vi "Server_Main.vi"() -> ()   [LabVIEW 2018, in "Cloud Server.lvlib"]
uses:
  Cloud Server.lvlib
  <vilib>/Platform/TimedLoop/XDataNode/timing_clust.ctl
  <vilib>/Platform/TimedLoop/XDataNode/nitl_modes.ctl
  <vilib>/Platform/TimedLoop/XDataNode/wakeup.ctl
  Data Def/Server_Error Handle Method.ctl
  Data Def/Server_Main Update Data.ctl
  Com VIs/Data Def/Data File Format.ctl
  Data Def/Server_Main Loop Queue Data.ctl
  Data Def/Server_Main Loop State.ctl
  Com VIs/Data Def/User Data.ctl
  Data Def/Server_Connection Manager Method.ctl
  Data Def/Server_Server Write Queue Data.ctl
  <vilib>/Platform/TimedLoop/XDataNode/XDataNode.xnode
  <vilib>/Platform/TimedLoop/XDataNode/XDNodeRunTimeDep.lvlib
panel:
  out "Number Of Connections":i32
  in  "Tab Control":T1(tab)
  out "User Data":T2 {"Last Login Time" format="%<%x %.3X>T"}
  out "Remote Data":waveform(dbl)(graph)
  out "User Picture":T3(plugin-control)
  in  "Scrollbar":i32(c297)
  out "Training Result":string
  out "Training Data":waveform(dbl)(graph)
  in  "Data Query List":i32(listbox)
  out "Query Data":waveform(dbl)(graph)
  in  "User Name List":i32(listbox)=-1
  # "Smart ECG Server"
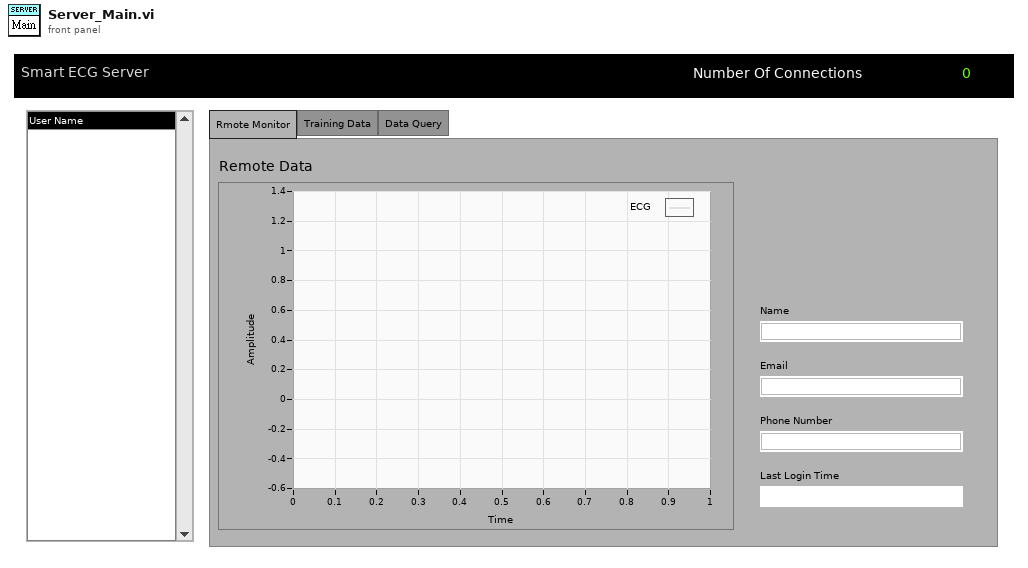
[diagram p1: front panel]
types:
  T1 = enum32{"Rmote Monitor", "Training Data", "Data Query"}
  T2 = cluster{"Name":string, "Email":string, "Phone Number":string, "Last Login Time":timestamp}
  T3 = typedef "IMAQ Image.ctl" = refnum<image>
  T4 = typedef "XDNodeRunTimeDep.lvlib/timing_clust.ctl" = cluster{"Expected End [f-1]":u64, "Actual End [f-1]":u64, "Finished Late? [f-1]":bool, "Expected End [i-1]":u64, "Actual End [i-1]":u64, "Finished Late? [i-1]":bool, "Expected Start [i]":u64, "Actual Start [i]":u64, "Expected Start [f]":u64, "Actual Start [f]":u64, "Source Name":string, "Structure Name":string, "Period":i64, "Deadline":i64, "Offset":i64, "Start":i64, "Priority":i32, "Timeout":i32, "Mode":T5, "Wakeup Reason":T6, "Error":errorcluster, "Source Type":string, "Secondary Source Type":string, "Global End Time":u64, "Global Start Time":u64, "Frame Duration":u64, "Iteration Duration":u64, "Assigned CPU":i32, "I/O Scan Engine Mode":u32}
  T5 = typedef "XDNodeRunTimeDep.lvlib/nitl_modes.ctl" = enum32{"No Change", "Process missed periods, maintain original phase", "Discard missed periods, maintain original phase", "Process missed periods, ignore original phase", "Discard missed periods, ignore original phase"}
  T6 = typedef "XDNodeRunTimeDep.lvlib/wakeup.ctl" = enum32{"Normal", "Aborted", "Asynchronous wakeup", "Timing source error", "Timed loop error", "Timeout"}
  T7 = typedef "Cloud Server.lvlib/Server_Main Loop Queue Data.ctl" = cluster{"Main Loop State":T8, "Data":variant}
  T8 = typedef "Cloud Server.lvlib/Server_Main Loop State.ctl" = enum16{"Detect", "Save", "Training", "Refresh User Name", "Stop"}
  T9 = typedef "User Data.ctl" = cluster{"Name":string, "Email":string, "Phone Number":string, "User Picture":u32[][], "Last Login Time":timestamp}
  T10 = typedef "Cloud Server.lvlib/Server_Main Data.ctl" = cluster{"Main VI Ref.":refnum<vi>, "Listener ID":refnum<k5>, "Meta data":T11[], "Main Queue":T13, "User Picture":T3}
  T11 = typedef "stm_MetaElement.ctl" = cluster{"Name":T12}
  T12 = typedef "stm_MetaDataElement.ctl" = string
  T13 = typedef "Cloud Server.lvlib/Server_Main Queue.ctl" = cluster{"Server Write Queue":refnum<queue>, "Main Loop Queue":refnum<queue>}
  T14 = typedef "Cloud Server.lvlib/Server_Server Write Queue Data.ctl" = cluster{"connection ID":refnum<k5>, "Meta Data":string, "Data":variant}
  T15 = typedef "User Registering Status.ctl" = enum16{"Failed", "Duplicate", "Success"}
  T16 = typedef "Cloud Server.lvlib/Server_Error Handle Method.ctl" = enum16{"Initialize", "Get Queue Ref.", "Enqueue", "Insert", "Flush", "Release"}
  T17 = typedef "Cloud Server.lvlib/Server_Connection Manager Method.ctl" = enum16{"Initialize", "Add", "Get", "Set Properties", "Get Properties", "Close", "Release"}
  T18 = typedef "Cloud Server.lvlib/Server_Main Update Data.ctl" = cluster{"Data":waveform(dbl), "connection ID":refnum<k5>}
  T19 = typedef "Cloud Server.lvlib/Server_Connection Properties.ctl" = cluster{"User Data":T9, "Data":waveform(dbl)}
  T20 = typedef "Data File Format.ctl" = cluster{"Data":waveform(dbl), "Abnormal?":bool, "Measure Time":timestamp, "User Name":string}
  T21 = typedef "Cloud Server.lvlib/Server_Training Data.ctl" = cluster{"Data":waveform(dbl), "Abnormal?":bool}
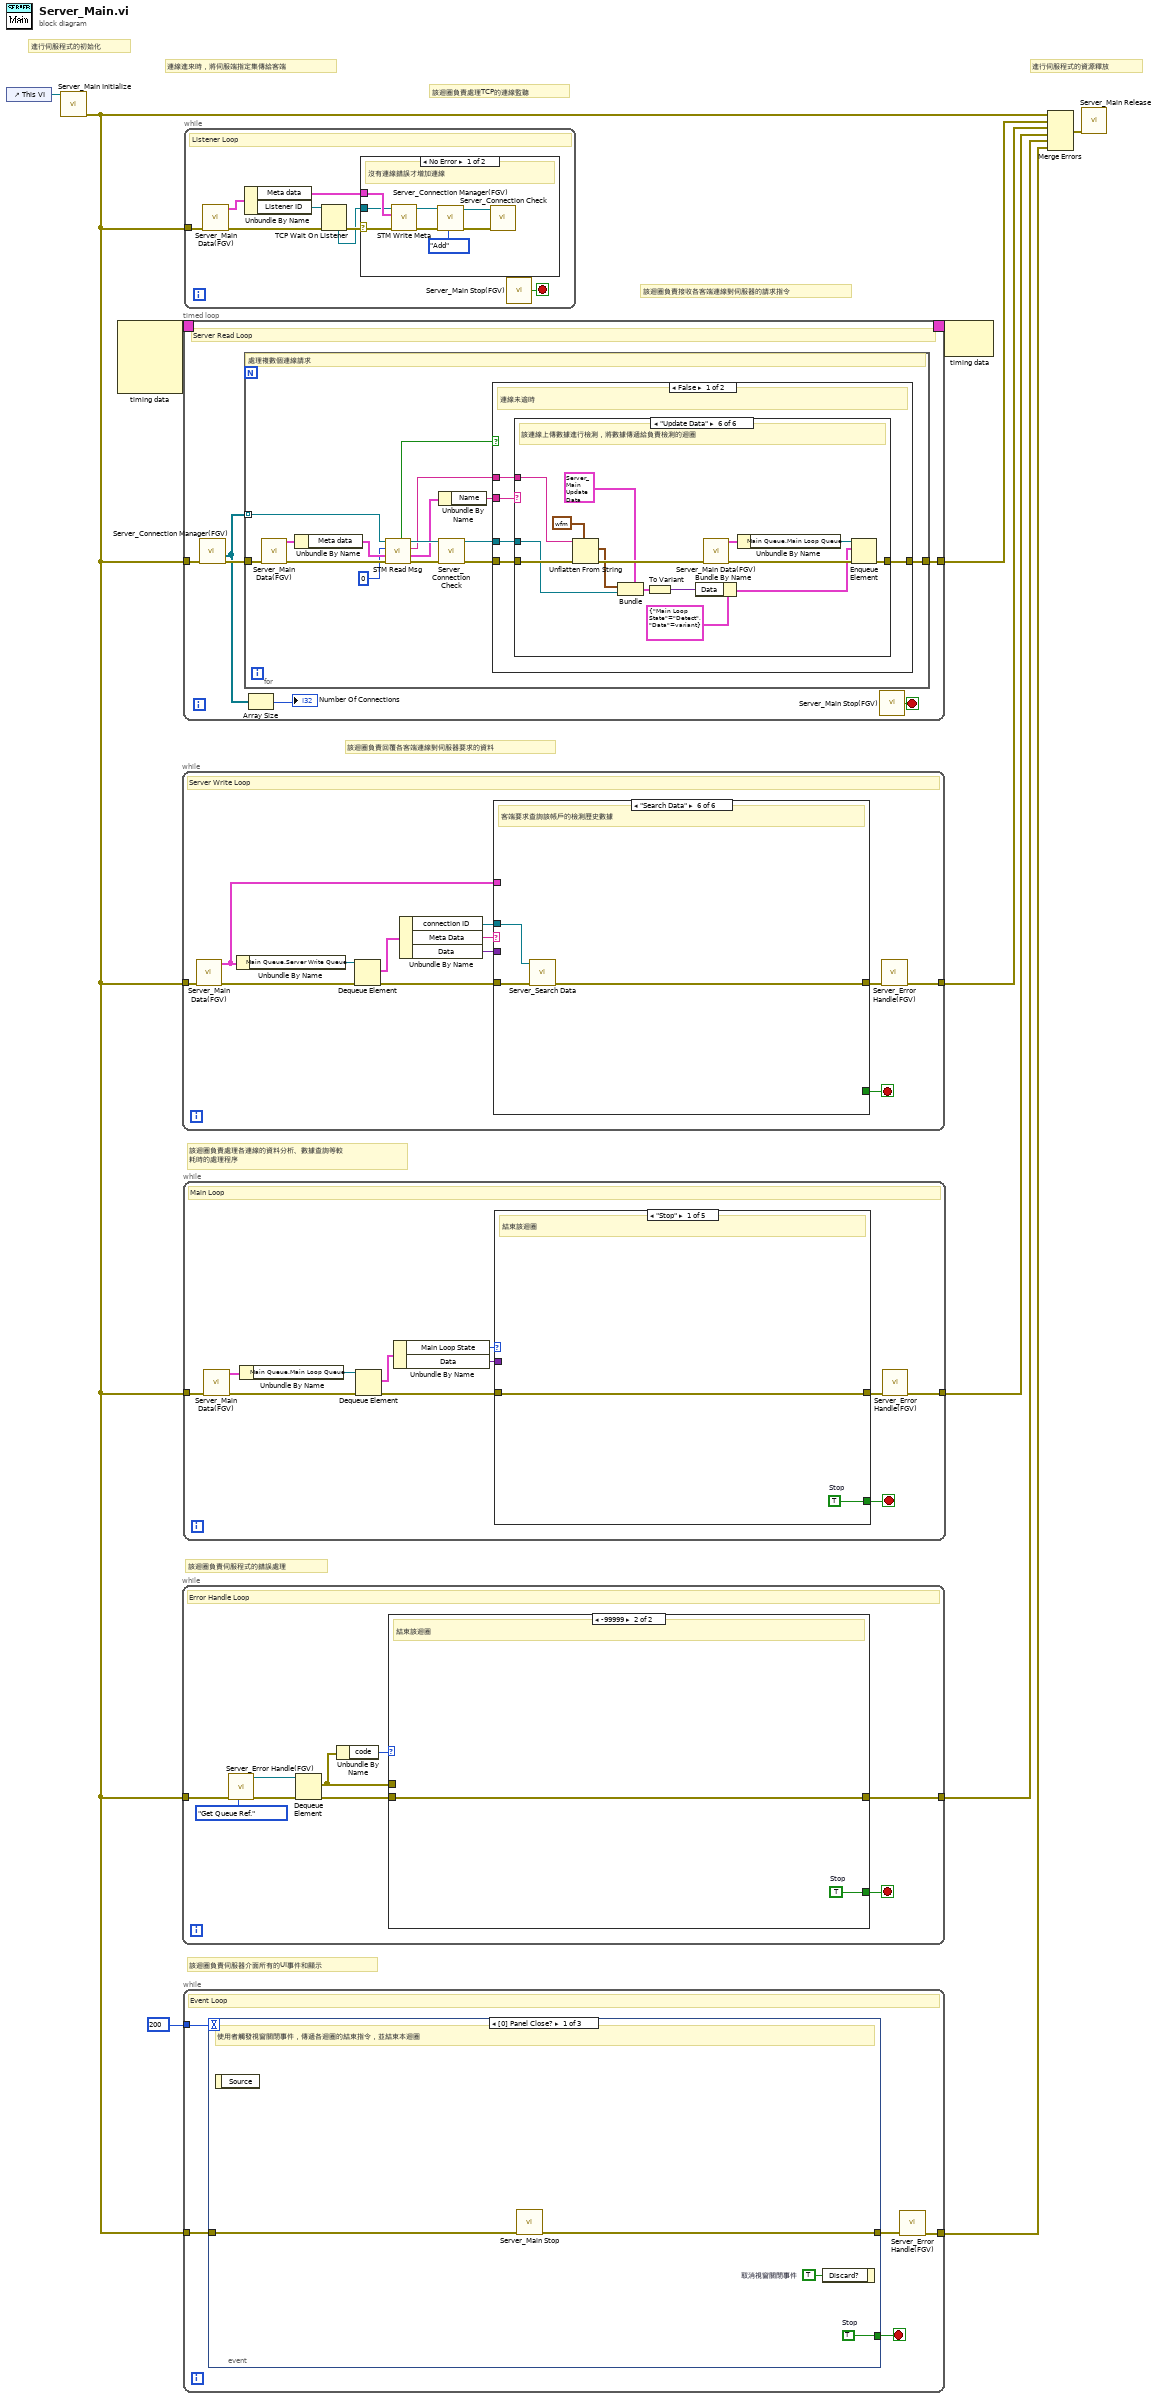
[diagram p0: block diagram]
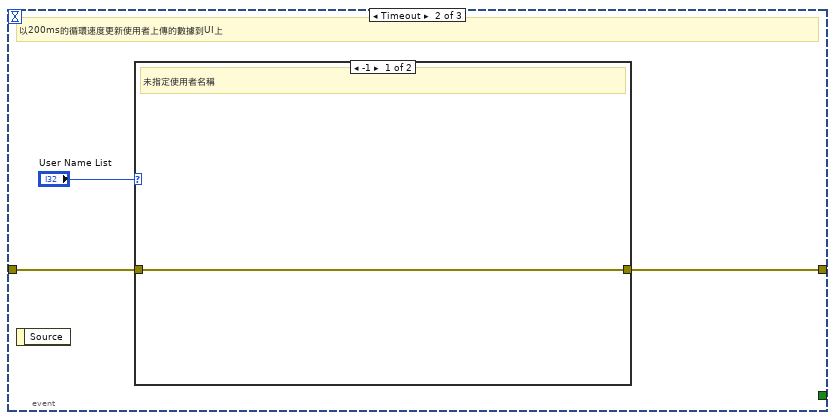
[diagram p2: hidden frame]
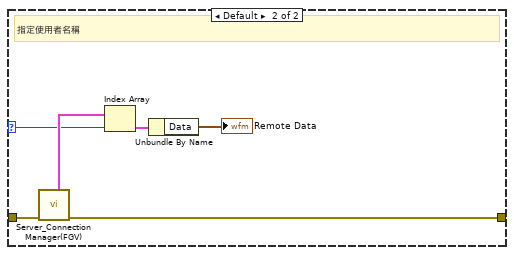
[diagram p3: hidden frame]
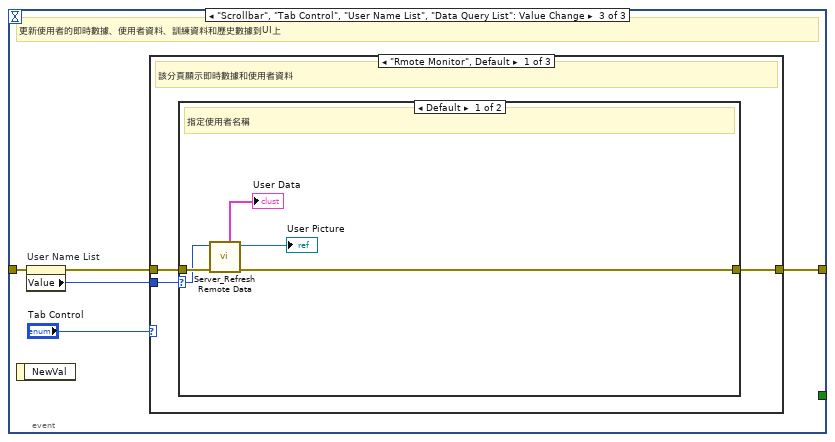
[diagram p4: hidden frame]
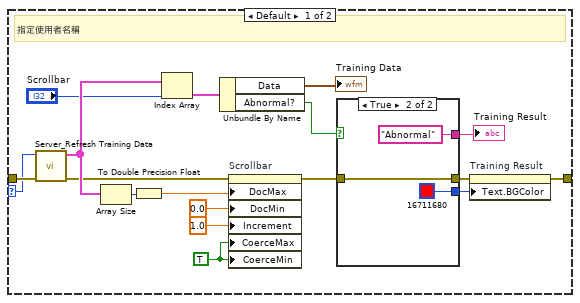
[diagram p7: hidden frame]
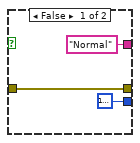
[diagram p8: hidden frame]
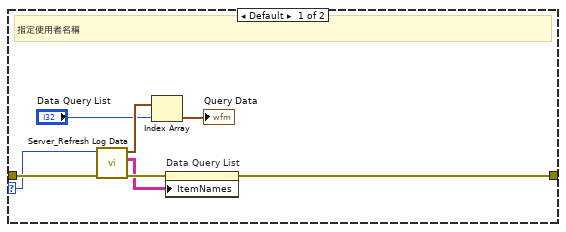
[diagram p10: hidden frame]
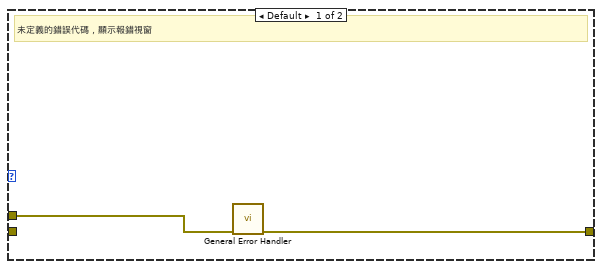
[diagram p11: hidden frame]
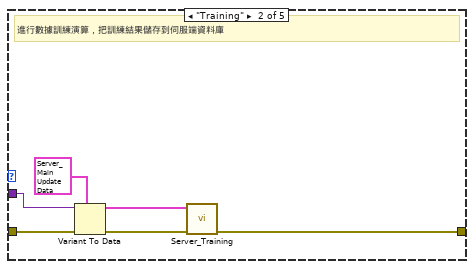
[diagram p12: hidden frame]
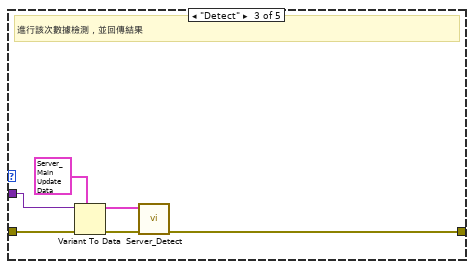
[diagram p13: hidden frame]
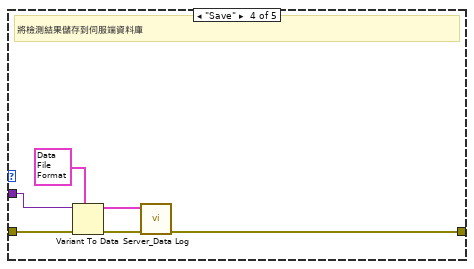
[diagram p14: hidden frame]
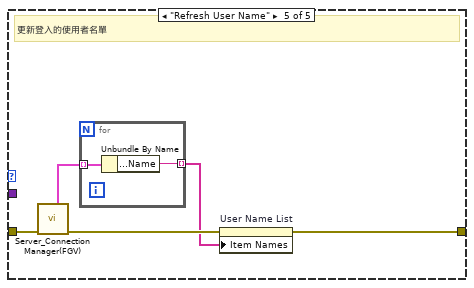
[diagram p15: hidden frame]
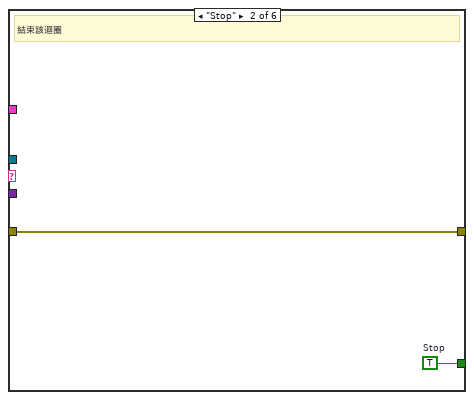
[diagram p17: hidden frame]
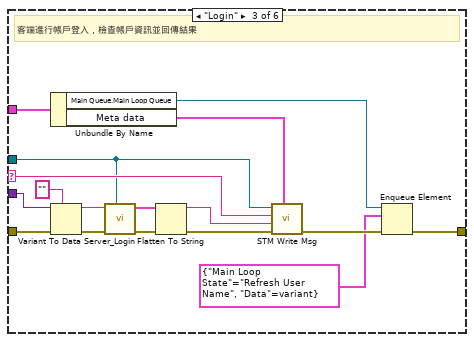
[diagram p18: hidden frame]
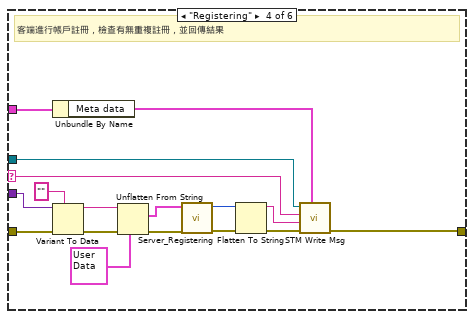
[diagram p19: hidden frame]
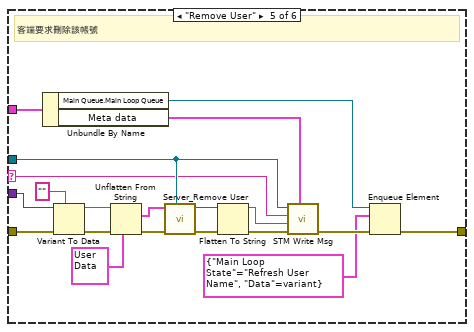
[diagram p20: hidden frame]
diagram:
  # "連線進來時，將伺服端指定集傳給客端"
  # "進行伺服程式的資源釋放"
  # "進行伺服程式的初始化"
  # "該迴圈負責伺服器介面所有的UI事件和顯示"
  # "該迴圈負責伺服程式的錯誤處理"
  # "該迴圈負責處理各連線的資料分析、數據查詢等較\n耗時的處理程序"
  # "該迴圈負責回覆各客端連線對伺服器要求的資料"
  # "該迴圈負責接收各客端連線對伺服器的請求指令"
  # "該迴圈負責處理TCP的連線監聽"
  n1 = control-ref of="This VI"() -> (w11:refnum<vi>)
  n2 = call "Server_Main Initialize.vi"("VI Reference"=w11) -> ("error out"=w3:errorcluster)  [unwired: 10 in]
  n3 = node-c288() -> (w10:T4)  [unwired: 4 in]
  n4 = while {
    tunnel: w3 -> [w23]
    tunnel: [w15] -> w6
    stop <- w13 stop-if-true
    # "Server Write Loop"
    n5 = call "Server_Main Data(FGV).vi"("error in"=w23) -> ("error out"=w22:errorcluster, "Main Data Out"=w12:T10)  [unwired: 9 in]
    n6 = Unbundle By Name(w12) -> ("Main Queue.Server Write Queue"=w21:refnum<queue>)
    n7 = Dequeue Element(queue=w21, error in (no error)=w22) -> (element=w20:T14, error out=w19:errorcluster)  [unwired: 1 in, 2 out]
    n8 = Unbundle By Name(w20) -> ("connection ID"=w16:refnum<k5>, "Meta Data"=w18:string, "Data"=w17:variant)
    n9 = case shown="\"Search Data\"" w18 {
      selector: w18 -> [_ _ w32 w51 w66 _]
      tunnel: w19 -> [w24 w26 w43 w60 w76 w83]
      tunnel: w17 -> [_ _ w42 w59 w75 _]
      tunnel: w16 -> [_ _ w31 w44 w68 w82]
      tunnel: [w24 w26 w29 w55 w63 w81] -> w14
      tunnel: [_ w25 _ _ _ _] -> w13
      tunnel: w12 -> [_ _ w38 w54 w70 _]
      frame Default {
        # "忽略，未定義的命令"
      }
      frame "Stop" {
        w25 = TRUE  # Stop
        # "結束該迴圈"
      }
      frame "Login" {
        # "客端進行帳戶登入，檢查帳戶資訊並回傳結果"
        n10 = Unbundle By Name(w38) -> ("Main Queue.Main Loop Queue"=w28:refnum<queue>, "Meta data"=w34:T11[])
        n11 = Variant To Data(error in=w43, type="", Variant=w42) -> (data=w39:string, error out=w40:errorcluster)
        n12 = call "Server_Login.vi"("connection ID"=w31, "error in"=w40, "User Name"=w39) -> ("error out"=w37:errorcluster, "User Data"=w36:T9)  [unwired: 7 in]
        n13 = Flatten To String(anything=w36, error in (no error)=w37) -> (data string=w33:string, error out=w35:errorcluster)  [unwired: 2 in, 1 out]
        n14 = call "STM Write Msg.vi"("Meta data"=w34, "error in (no error)"=w35, "Data"=w33, "Name"=w32, "connection ID"=w31) -> ("error out"=w30:errorcluster)  [unwired: 5 in, 1 out]
        n15 = Enqueue Element(queue=w28, element=T7 {"Main Loop State"=enum."Refresh User Name", "Data"=variant}, error in (no error)=w30) -> (error out=w29:errorcluster)  [unwired: 1 in, 2 out]
      }
      frame "Registering" {
        # "客端進行帳戶註冊，檢查有無重複註冊，並回傳結果"
        n16 = Unbundle By Name(w54) -> ("Meta data"=w53:T11[])
        n17 = Variant To Data(error in=w60, type="", Variant=w59) -> (data=w48:string, error out=w49:errorcluster)
        n18 = Unflatten From String(type=T9 {"Name"="Guset", "Email"="", "Phone Number"="", "User Picture"=array225x225[50625 elements], "Last Login Time"=timestamp(0 s since 1904-01-01)} ("User Data"), binary string=w48, error in (no error)=w49) -> (value=w45:T9, error out=w46:errorcluster)  [unwired: 2 in, 1 out]
        n19 = call "Server_Registering.vi"("error in"=w46, "User Data"=w45) -> ("error out"=w58:errorcluster, "User Registering Status"=w57:T15)  [unwired: 8 in]
        n20 = Flatten To String(anything=w57, error in (no error)=w58) -> (data string=w52:string, error out=w56:errorcluster)  [unwired: 2 in, 1 out]
        n21 = call "STM Write Msg.vi"("Meta data"=w53, "error in (no error)"=w56, "Data"=w52, "Name"=w51, "connection ID"=w44) -> ("error out"=w55:errorcluster)  [unwired: 5 in, 1 out]
      }
      frame "Remove User" {
        # "客端要求刪除該帳號"
        n22 = Unbundle By Name(w70) -> ("Main Queue.Main Loop Queue"=w62:refnum<queue>, "Meta data"=w69:T11[])
        n23 = Variant To Data(error in=w76, type="", Variant=w75) -> (data=w78:string, error out=w79:errorcluster)
        n24 = Unflatten From String(type=T9 {"Name"="Guset", "Email"="", "Phone Number"="", "User Picture"=array225x225[50625 elements], "Last Login Time"=timestamp(0 s since 1904-01-01)} ("User Data"), binary string=w78, error in (no error)=w79) -> (value=w73:T9, error out=w74:errorcluster)  [unwired: 2 in, 1 out]
        n25 = call "Server_Remove User.vi"("connection ID"=w68, "error in"=w74, "User Data"=w73) -> ("error out"=w72:errorcluster, "OK?"=w71:bool)  [unwired: 7 in]
        n26 = Flatten To String(anything=w71, error in (no error)=w72) -> (data string=w65:string, error out=w67:errorcluster)  [unwired: 2 in, 1 out]
        n27 = call "STM Write Msg.vi"("Meta data"=w69, "error in (no error)"=w67, "Data"=w65, "Name"=w66, "connection ID"=w68) -> ("error out"=w64:errorcluster)  [unwired: 5 in, 1 out]
        n28 = Enqueue Element(queue=w62, element=T7 {"Main Loop State"=enum."Refresh User Name", "Data"=variant}, error in (no error)=w64) -> (error out=w63:errorcluster)  [unwired: 1 in, 2 out]
      }
      frame "Search Data" {
        # "客端要求查詢該帳戶的檢測歷史數據"
        n29 = call "Server_Search Data.vi"("error in"=w83, "connection ID"=w82) -> ("error out"=w81:errorcluster)  [unwired: 9 in]
      }
    }
    n30 = call "Server_Error Handle(FGV).vi"("error in"=w14) -> ("error out"=w15:errorcluster)  [unwired: 9 in, 1 out]
  }
  n31 = while {
    tunnel: w3 -> [w90]
    tunnel: [w85] -> w4
    stop <- w91 stop-if-true
    # "Error Handle Loop"
    n32 = call "Server_Error Handle(FGV).vi"("Error Handle Method(Enqueue)"=Server_Error_Handle_Method."Get Queue Ref.", "error in"=w90) -> ("error out"=w89:errorcluster, "Queue Ref."=w87:refnum<queue>)  [unwired: 8 in]
    n33 = Dequeue Element(queue=w87, error in (no error)=w89) -> (element=w84:errorcluster, error out=w92:errorcluster)  [unwired: 1 in, 2 out]
    n34 = Unbundle By Name(w84) -> ("code"=w86:i32)
    n35 = case shown="-99999" w86 {
      tunnel: w92 -> [_ w95]
      tunnel: [w94 w95] -> w85
      tunnel: [_ w96] -> w91
      tunnel: w84 -> [w93 _]
      frame Default {
        # "未定義的錯誤代碼，顯示報錯視窗"
        n36 = call <vilib>:"General Error Handler.vi"("error in (no error)"=w93) -> ("error out"=w94:errorcluster)  [unwired: 10 in, 4 out]
      }
      frame -99999 {
        w96 = TRUE  # Stop
        # "結束該迴圈"
      }
    }
  }
  n37 = timed-loop {
    tunnel: w3 -> [w102]
    timing: w10 -> [_]
    timing-out: [_] -> w9
    tunnel: [w99] -> w8
    stop <- w100 stop-if-true
    # "Server Read Loop"
    n38 = call "Server_Connection Manager(FGV).vi"("error in"=w102) -> ("error out"=w101:errorcluster, "All Connections"=w98:refnum<k5>[])  [unwired: 6 in, 3 out]
    n39 = for {
      tunnel: w101 -> [w114]
      tunnel: w98 -> [w117] mode=indexing
      tunnel: [w104] -> w99
      # "處理複數個連線請求"
      n40 = call "Server_Main Data(FGV).vi"("error in"=w114) -> ("error out"=w112:errorcluster, "Main Data Out"=w113:T10)  [unwired: 9 in]
      n41 = Unbundle By Name(w113) -> ("Meta data"=w111:T11[])
      n42 = call "STM Read Msg.vi"("error in"=w112, "Meta data"=w111, "timeout ms (25000)"=0, "connection ID"=w117) -> ("error out"=w116:errorcluster, "Meta element"=w106:T11, "data string"=w107:string, "connection ID out"=w115:refnum<k5>, "Timed Out?"=w103:bool)  [unwired: 2 in, 1 out]
      n43 = Unbundle By Name(w106) -> ("Name"=w105:T12)
      n44 = call "Server_Connection Check.vi"("error in"=w116, "Connection In"=w115) -> ("error out"=w109:errorcluster, "Connection out"=w108:refnum<k5>)  [unwired: 7 in, 1 out]
      n45 = case shown="False" w103 {
        tunnel: w109 -> [w120 w187]
        tunnel: w108 -> [w118 _]
        tunnel: w107 -> [w122 _]
        tunnel: w105 -> [w121 _]
        tunnel: [w119 w187] -> w104
        frame False {
          # "連線未逾時"
          n46 = case shown="\"Update Data\"" w121 {
            selector: w121 -> [_ w127 _ _ _ _]
            tunnel: w122 -> [_ w129 _ w155 w169 w184]
            tunnel: w120 -> [w123 w134 w143 w156 w170 w185]
            tunnel: [w123 w124 w136 w145 w164 w179] -> w119
            tunnel: w118 -> [_ w126 w141 w152 w167 w182]
            frame Default {
              # "忽略，未定義的命令"
            }
            frame "Login", "Registering", "Remove User", "Search Data" {
              # "把請求傳遞到負責TCP回復資料的迴圈"
              n47 = To Variant(anything=w129) -> (Variant=w128:variant)
              n48 = call "Server_Main Data(FGV).vi"("error in"=w134) -> ("error out"=w132:errorcluster, "Main Data Out"=w133:T10)  [unwired: 9 in]
              n49 = Unbundle By Name(w133) -> ("Main Queue.Server Write Queue"=w131:refnum<queue>)
              n50 = Bundle By Name(cluster=T14 {"connection ID"=refnum, "Meta Data"="", "Data"=variant} ("element"), "Data"=w128, "Meta Data"=w127, "connection ID"=w126) -> (w125:T14)
              n51 = Enqueue Element(queue=w131, element=w125, error in (no error)=w132) -> (error out=w124:errorcluster)  [unwired: 1 in, 2 out]
            }
            frame "Logout" {
              # "該連線進行登出"
              n52 = call "Server_Connection Manager(FGV).vi"("Connection Manager Method(Get)"=Server_Connection_Manager_Method."Close", "error in"=w143, "Connection In"=w141) -> ("error out"=w140:errorcluster)  [unwired: 4 in, 4 out]
              n53 = call "Server_Main Data(FGV).vi"("error in"=w140) -> ("error out"=w138:errorcluster, "Main Data Out"=w139:T10)  [unwired: 9 in]
              n54 = Unbundle By Name(w139) -> ("Main Queue.Main Loop Queue"=w137:refnum<queue>)
              n55 = Enqueue Element(queue=w137, element=T7 {"Main Loop State"=enum."Refresh User Name", "Data"=variant}, error in (no error)=w138) -> (error out=w136:errorcluster)  [unwired: 1 in, 2 out]
            }
            frame "Live Mode" {
              # "該連線連續上傳資料"
              n56 = Unflatten From String(type=waveform(dbl) {"t0"=timestamp(0 s since 1904-01-01), "dt"=1.0, "Y"=[]} ("waveform"), binary string=w155, error in (no error)=w156) -> (value=w146:waveform(dbl), error out=w153:errorcluster)  [unwired: 2 in, 1 out]
              n57 = call "Server_Connection Manager(FGV).vi"("Connection Manager Method(Get)"=Server_Connection_Manager_Method."Get Properties", "error in"=w153, "Connection In"=w152) -> ("error out"=w150:errorcluster, "Connection Properties Out"=w147:T19, "Connection Out"=w149:refnum<k5>)  [unwired: 4 in, 2 out]
              n58 = Bundle By Name(cluster=w147, "Data"=w146) -> (w144:T19)
              n59 = call "Server_Connection Manager(FGV).vi"("Connection Manager Method(Get)"=Server_Connection_Manager_Method."Set Properties", "error in"=w150, "Connection Properties In"=w144, "Connection In"=w149) -> ("error out"=w145:errorcluster)  [unwired: 3 in, 4 out]
            }
            frame "Training" {
              # "該連線進行訓練演算，將資料傳遞給負責演算的迴圈"
              n60 = Unflatten From String(type=waveform(dbl) {"t0"=timestamp(0 s since 1904-01-01), "dt"=1.0, "Y"=[]} ("Data"), binary string=w169, error in (no error)=w170) -> (value=w157:waveform(dbl), error out=w168:errorcluster)  [unwired: 2 in, 1 out]
              n61 = Bundle(cluster=T18 {"Data"={"t0"=timestamp(0 s since 1904-01-01), "dt"=1.0, "Y"=[]}, "connection ID"=refnum} ("Main Training Data"), "Data"=w157, "connection ID"=w167) -> (w163:T18)
              n62 = To Variant(anything=w163) -> (Variant=w162:variant)
              n63 = Bundle By Name(cluster=T7 {"Main Loop State"=enum."Training", "Data"=variant} ("element"), "Data"=w162) -> (w160:T7)
              n64 = call "Server_Main Data(FGV).vi"("error in"=w168) -> ("error out"=w166:errorcluster, "Main Data Out"=w171:T10)  [unwired: 9 in]
              n65 = Unbundle By Name(w171) -> ("Main Queue.Main Loop Queue"=w165:refnum<queue>)
              n66 = Enqueue Element(queue=w165, element=w160, error in (no error)=w166) -> (error out=w164:errorcluster)  [unwired: 1 in, 2 out]
            }
            frame "Update Data" {
              # "該連線上傳數據進行檢測，將數據傳遞給負責檢測的迴圈"
              n67 = Unflatten From String(type=waveform(dbl) {"t0"=timestamp(0 s since 1904-01-01), "dt"=1.0, "Y"=[]} ("Data"), binary string=w184, error in (no error)=w185) -> (value=w172:waveform(dbl), error out=w183:errorcluster)  [unwired: 2 in, 1 out]
              n68 = Bundle(cluster=T18 {"Data"={"t0"=timestamp(0 s since 1904-01-01), "dt"=1.0, "Y"=[]}, "connection ID"=refnum} ("Main Training Data"), "Data"=w172, "connection ID"=w182) -> (w178:T18)
              n69 = To Variant(anything=w178) -> (Variant=w177:variant)
              n70 = Bundle By Name(cluster=T7 {"Main Loop State"=enum."Detect", "Data"=variant} ("element"), "Data"=w177) -> (w175:T7)
              n71 = call "Server_Main Data(FGV).vi"("error in"=w183) -> ("error out"=w181:errorcluster, "Main Data Out"=w186:T10)  [unwired: 9 in]
              n72 = Unbundle By Name(w186) -> ("Main Queue.Main Loop Queue"=w180:refnum<queue>)
              n73 = Enqueue Element(queue=w180, element=w175, error in (no error)=w181) -> (error out=w179:errorcluster)  [unwired: 1 in, 2 out]
            }
          }
        }
        frame True {
          # "逾時，沒收到請求"
        }
      }
    }
    n74 = Array Size(array=w98) -> (size(s)=→"Number Of Connections":i32)
    n75 = call "Server_Main Stop(FGV).vi"() -> ("Stop Out"=w100:bool)  [unwired: 4 in]
  }
  n76 = while {
    tunnel: w3 -> [w200]
    tunnel: [w192] -> w5
    stop <- w190 stop-if-true
    # "Main Loop"
    n77 = call "Server_Main Data(FGV).vi"("error in"=w200) -> ("error out"=w198:errorcluster, "Main Data Out"=w199:T10)  [unwired: 9 in]
    n78 = Unbundle By Name(w199) -> ("Main Queue.Main Loop Queue"=w197:refnum<queue>)
    n79 = Dequeue Element(queue=w197, error in (no error)=w198) -> (element=w196:T7, error out=w195:errorcluster)  [unwired: 1 in, 2 out]
    n80 = Unbundle By Name(w196) -> ("Main Loop State"=w194:T8, "Data"=w193:variant)
    n81 = case shown="\"Stop\"" w194 {
      tunnel: w195 -> [w202 w208 w214 w220 w225]
      tunnel: w193 -> [_ w207 w213 w219 _]
      tunnel: [w202 w204 w209 w217 w221] -> w191
      tunnel: [w201 _ _ _ _] -> w190
      frame "Stop" {
        w201 = TRUE  # Stop
        # "結束該迴圈"
      }
      frame "Training" {
        # "進行數據訓練演算，把訓練結果儲存到伺服端資料庫"
        n82 = Variant To Data(error in=w208, type=T18 {"Data"={"t0"=timestamp(0 s since 1904-01-01), "dt"=1.0, "Y"=[]}, "connection ID"=refnum} ("Main Training Data"), Variant=w207) -> (data=w203:T18, error out=w205:errorcluster)
        n83 = call "Server_Training.vi"("error in"=w205, "Main Update Data"=w203) -> ("error out"=w204:errorcluster)  [unwired: 9 in]
      }
      frame "Detect" {
        # "進行該次數據檢測，並回傳結果"
        n84 = Variant To Data(error in=w214, type=T18 {"Data"={"t0"=timestamp(0 s since 1904-01-01), "dt"=1.0, "Y"=[]}, "connection ID"=refnum} ("Main Training Data"), Variant=w213) -> (data=w210:T18, error out=w211:errorcluster)
        n85 = call "Server_Detect.vi"("error in"=w211, "Main Update Data"=w210) -> ("error out"=w209:errorcluster)  [unwired: 9 in]
      }
      frame "Save" {
        # "將檢測結果儲存到伺服端資料庫"
        n86 = Variant To Data(error in=w220, type=T20 {"Data"={"t0"=timestamp(0 s since 1904-01-01), "dt"=1.0, "Y"=[]}, "Abnormal?"=FALSE, "Measure Time"=timestamp(0 s since 1904-01-01), "User Name"=""} ("Data File Format"), Variant=w219) -> (data=w216:T20, error out=w218:errorcluster)
        n87 = call "Server_Data Log.vi"("error in"=w218, "Data File Format"=w216) -> ("error out"=w217:errorcluster)  [unwired: 9 in]
      }
      frame "Refresh User Name" {
        # "更新登入的使用者名單"
        n88 = call "Server_Connection Manager(FGV).vi"("error in"=w225) -> ("error out"=w223:errorcluster, "All Connection Properties"=w224:T19[])  [unwired: 6 in, 3 out]
        n89 = for {
          tunnel: w224 -> [w227] mode=indexing
          tunnel: [w226] -> w222 mode=indexing
          n90 = Unbundle By Name(w227) -> ("User Data.Name"=w226:string)
        }
        n91 = property on="User Name List" class="LstBox (strict)"(error in=w223, "Item Names"=w222) -> (error out=w221:errorcluster)  [unwired: 1 in, 1 out]
      }
    }
    n92 = call "Server_Error Handle(FGV).vi"("error in"=w191) -> ("error out"=w192:errorcluster)  [unwired: 9 in, 1 out]
  }
  n93 = while {
    tunnel: w3 -> [w232]
    tunnel: [w231] -> w2
    tunnel: 200 -> [w228]
    stop <- w230 stop-if-true
    # "Event Loop"
    n94 = event shown="[0] Panel Close?" {
      selector: _ -> [_ _ _]
      dyn-events: _ -> [_ _ _]
      timeout: w228 -> [_ _ _]
      tunnel: w232 -> [w234 w239 w250]
      tunnel: [w236 _ _] -> w230
      tunnel: [w233 w237 w247] -> w229
      event Panel Close? {
        w235 = TRUE  # 取消視窗關閉事件
        w236 = TRUE  # Stop
        # "使用者觸發視窗關閉事件，傳遞各迴圈的結束指令，並結束本迴圈"
        n95 = event-data() -> ()  [unwired: 1 in, 1 out]
        n96 = call "Server_Main Stop.vi"("error in"=w234) -> ("error out"=w233:errorcluster)  [unwired: 10 in]
        n97 = event-data("Discard?"=w235) -> ()  [unwired: 1 in, 1 out]
      }
      event Timeout {
        # "以200ms的循環速度更新使用者上傳的數據到UI上"
        n98 = event-data() -> ()  [unwired: 1 in, 1 out]
        n99 = case shown="-1" "User Name List" {
          selector: "User Name List" -> [_ w244]
          tunnel: w239 -> [w240 w246]
          tunnel: [w240 w242] -> w237
          frame -1 {
            # "未指定使用者名稱"
          }
          frame Default {
            # "指定使用者名稱"
            n100 = call "Server_Connection Manager(FGV).vi"("error in"=w246) -> ("error out"=w242:errorcluster, "All Connection Properties"=w245:T19[])  [unwired: 6 in, 3 out]
            n101 = Index Array(array=w245, index=w244) -> (element=w243:T19)
            n102 = Unbundle By Name(w243) -> ("Data"=→"Remote Data":waveform(dbl))
          }
        }
      }
      event "Scrollbar", "Tab Control", "User Name List", "Data Query List": Value Change {
        # "更新使用者的即時數據、使用者資料、訓練資料和歷史數據到UI上"
        n103 = event-data() -> ()  [unwired: 1 in, 1 out]
        n104 = property on="User Name List" class="LstBox (strict)"(error in=w250) -> (error out=w249:errorcluster, "Value"=w248:i32)  [unwired: 1 in, 1 out]
        n105 = case shown="\"Rmote Monitor\", Default" "Tab Control" {
          tunnel: w249 -> [w253 w262 w291]
          tunnel: w248 -> [w254 w263 w290]
          tunnel: [w252 w261 w289] -> w247
          frame "Rmote Monitor", Default {
            # "該分頁顯示即時數據和使用者資料"
            n106 = case shown="Default" w254 {
              selector: w254 -> [w255 _]
              tunnel: w253 -> [w257 w260]
              tunnel: [w256 w260] -> w252
              frame Default {
                # "指定使用者名稱"
                n107 = call "Server_Refresh Remote Data.vi"("error in"=w257, "Index"=w255) -> ("error out"=w256:errorcluster, "Image"=→"User Picture":T3, "User Data"=→"User Data":T2)  [unwired: 7 in]
              }
              frame -1 {
                # "未指定使用者名稱"
              }
            }
          }
          frame "Training Data" {
            # "該分頁顯示使用者的訓練資料"
            n108 = case shown="-1" w263 {
              selector: w263 -> [w280 _]
              tunnel: w262 -> [w281 w288]
              tunnel: [w275 w288] -> w261
              frame Default {
                w264 = TRUE ("Coerce Minimum Value")
                # "指定使用者名稱"
                n109 = call "Server_Refresh Training Data.vi"("error in"=w281, "Index"=w280) -> ("error out"=w269:errorcluster, "Training Data"=w278:T21[])  [unwired: 8 in]
                n110 = Array Size(array=w278) -> (size(s)=w279:i32)
                n111 = To Double Precision Float(number=w279) -> (double precision float=w267:dbl)
                n112 = Index Array(array=w278, index="Scrollbar") -> (element=w277:T21)
                n113 = Unbundle By Name(w277) -> ("Data"=→"Training Data":waveform(dbl), "Abnormal?"=w274:bool)
                n114 = property on="Scrollbar" class="Scroll (strict)"(error in=w269, "DocMax"=w267, "DocMin"=0.0 ("Scale.Range:Minimum"), "Increment"=1.0, "CoerceMax"=w264, "CoerceMin"=w264) -> (error out=w268:errorcluster)  [unwired: 1 in, 1 out]
                n115 = case shown="True" w274 {
                  tunnel: w268 -> [w284 w287]
                  tunnel: [w284 w287] -> w273
                  tunnel: [u32 16777216 u32 16711680] -> w272
                  tunnel: ["Normal" "Abnormal"] -> w271
                  frame False {
                  }
                  frame True {
                  }
                }
                "Training Result" <- w271
                n116 = property on="Training Result" class="Str"(error in=w273, "Text.BGColor"=w272) -> (error out=w275:errorcluster)  [unwired: 1 in, 1 out]
              }
              frame -1 {
                # "未指定使用者名稱"
              }
            }
          }
          frame "Data Query" {
            # "該分頁顯示使用者的檢測歷史數據"
            n117 = case shown="-1" w290 {
              selector: w290 -> [w298 _]
              tunnel: w291 -> [w299 w300]
              tunnel: [w296 w300] -> w289
              frame Default {
                # "指定使用者名稱"
                n118 = call "Server_Refresh Log Data.vi"("error in"=w299, "Index"=w298) -> ("error out"=w297:errorcluster, "Data Query List"=w295:string[][], "Data"=w294:waveform(dbl)[])  [unwired: 7 in]
                n119 = Index Array(array=w294, index="Data Query List") -> (element=→"Query Data":waveform(dbl))
                n120 = property on="Data Query List" class="MCListbox (strict)"(error in=w297, "ItemNames"=w295) -> (error out=w296:errorcluster)  [unwired: 1 in, 1 out]
              }
              frame -1 {
                # "未指定使用者名稱"
              }
            }
          }
        }
      }
    }
    n121 = call "Server_Error Handle(FGV).vi"("error in"=w229) -> ("error out"=w231:errorcluster)  [unwired: 9 in, 1 out]
  }
  n122 = while {
    tunnel: w3 -> [w308]
    stop <- w303 stop-if-true
    # "Listener Loop"
    n123 = call "Server_Main Data(FGV).vi"("error in"=w308) -> ("error out"=w306:errorcluster, "Main Data Out"=w307:T10)  [unwired: 9 in]
    n124 = Unbundle By Name(w307) -> ("Meta data"=w302:T11[], "Listener ID"=w305:refnum<k5>)
    n125 = TCP Wait On Listener(8:w306, 11:w305) -> (0:w304:errorcluster, 4:w301:refnum<k5>)  [unwired: 2 in, 3 out]
    n126 = case shown="No Error" w304 {
      selector: w304 -> [w314 _]
      tunnel: w301 -> [w315 _]
      tunnel: w302 -> [w316 _]
      frame No Error {
        # "沒有連線錯誤才增加連線"
        n127 = call "STM Write Meta.vi"("error in"=w314, "Meta data"=w316, "connection ID"=w315) -> ("error out"=w310:errorcluster, "connection ID out"=w309:refnum<k5>)  [unwired: 7 in]
        n128 = call "Server_Connection Manager(FGV).vi"("Connection Manager Method(Get)"=Server_Connection_Manager_Method."Add", "error in"=w310, "Connection In"=w309) -> ("error out"=w312:errorcluster, "Connection Out"=w311:refnum<k5>)  [unwired: 4 in, 3 out]
        n129 = call "Server_Connection Check.vi"("error in"=w312, "Connection In"=w311) -> ()  [unwired: 7 in, 3 out]
      }
      frame Error {
        # "連線錯誤"
      }
    }
    n130 = call "Server_Main Stop(FGV).vi"() -> ("Stop Out"=w303:bool)  [unwired: 4 in]
  }
  n131 = node-c288(w9) -> ()  [unwired: 1 out]
  n132 = Merge Errors(w3, w8, w6, w5, w4, w2) -> (w7:errorcluster)
  n133 = call "Server_Main Release.vi"("error in"=w7) -> ()  [unwired: 10 in, 1 out]
